vi "Flow Settings Dialog.vi"(8 "error in (no error)":errorcluster, 11 "Flow Module Config In":T1={"GUID"="", "Drop Coords"={"Horizontal"=0, "Vertical"=0}, "Process Name"="", "Settings"={"Cycle Period"=500.0, "Bronkhorst M13"={"VISA resource name"="", "Simulated?"=FALSE}, "Flow Meter Type"="", "Bronkhorst M14"={"VISA resource name"="", "Simulated?"=FALSE}}, "Load Count"=0}) -> (0 "error out":errorcluster, 1 "Cancelled?":bool=TRUE, 2 "UI Refresh Needed?":bool, 3 "Flow Module Config Out":T1={"GUID"="", "Drop Coords"={"Horizontal"=0, "Vertical"=0}, "Process Name"="", "Settings"={"Cycle Period"=500.0, "Bronkhorst M13"={"VISA resource name"="", "Simulated?"=FALSE}, "Flow Meter Type"="", "Bronkhorst M14"={"VISA resource name"="", "Simulated?"=FALSE}}, "Load Count"=0})   [LabVIEW 2018, in "Flow Module.lvlib"]
doc: "Dialog for selecting user specified settings."
uses:
  Flow Module.lvlib
  Feed Module/Controls/Flow Module Settings Cluster.ctl
  Mettler Toledo/Controls/Settings Cluster.ctl
  Feed Module/Controls/Flow Module Config Cluster.ctl
  <vilib>/Utility/miscctls.llb/LVPoint32TypeDef.ctl
  <vilib>/Utility/xml.llb/Write to XML File(string).vi
  Settings/Settings.lvlib
  Bronkhorst M13 Flow Meter/Bronkhorst M13 Flow Meter.lvlib
  Bronkhorst M14 Flow Meter/Bronkhorst M14 Flow Meter.lvlib
  Mettler Toledo/Mettler Toledo.lvlib
panel:
  in  "Module Name":string
  in  "Flow Meter Configuration":T3={"Cycle Period"=500.0, "Bronkhorst M13"={"VISA resource name"="", "Simulated?"=FALSE}, "Flow Meter Type"="Default", "Bronkhorst M14"={"VISA resource name"="", "Simulated?"=FALSE}}
  in  "Cancel Button":bool
  in  "OK Button":bool
  # "Non visible portion of dialog (needed for connector pane)."
  # "Flow Meter Settings"
  # "Flow Meter Settings"
  # "Flow Meter Settings"
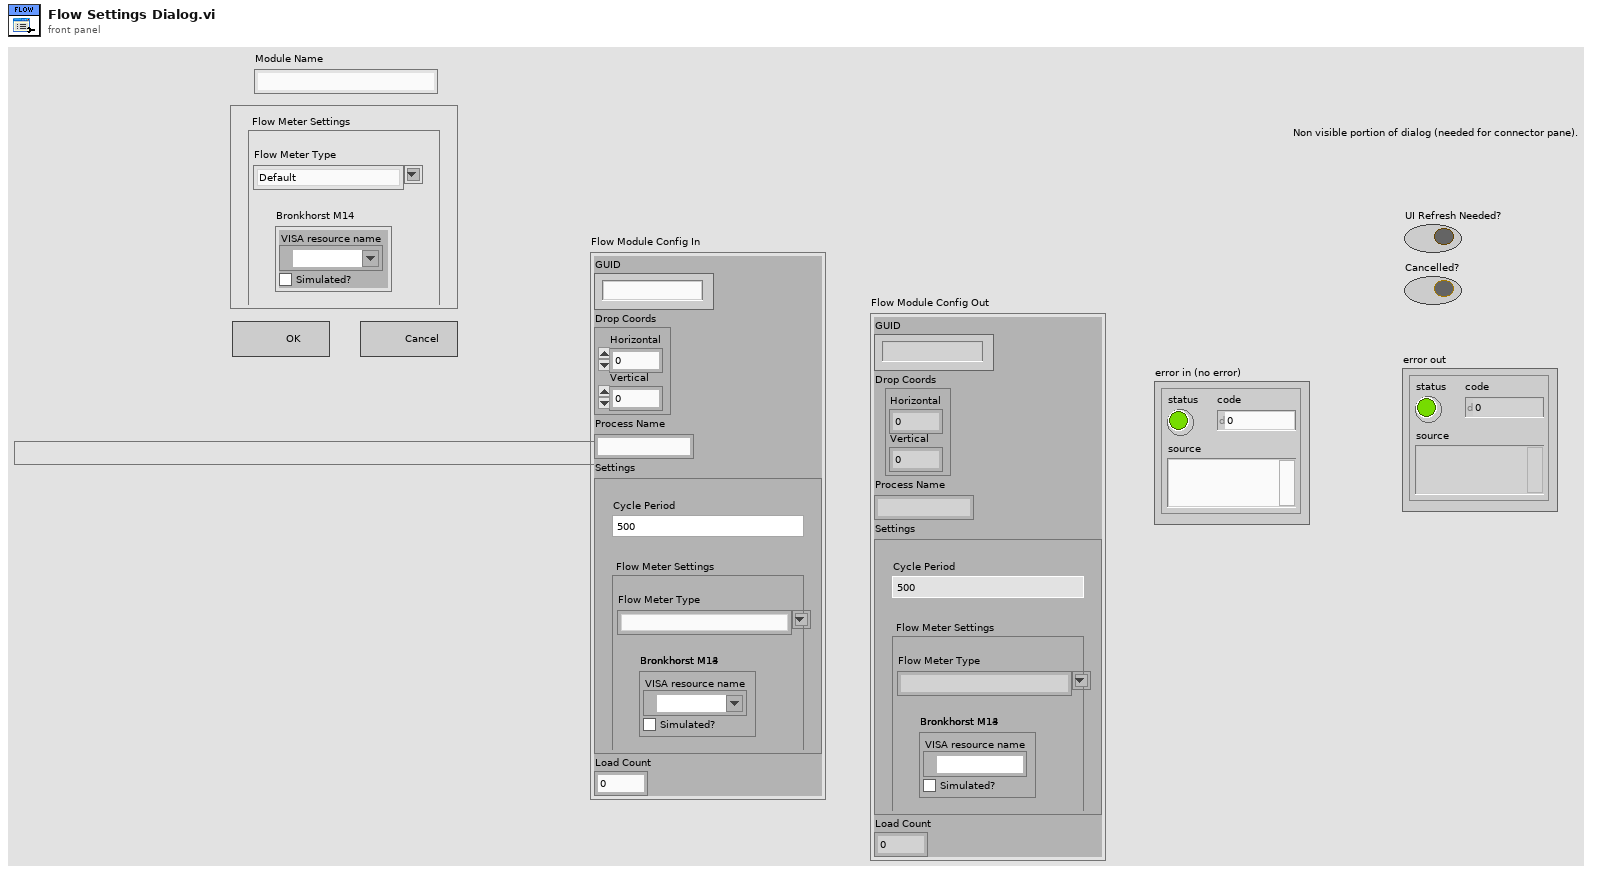
[diagram p1: front panel]
types:
  T1 = typedef "Flow Module.lvlib/Flow Module Config Cluster.ctl" = cluster{"GUID":string, "Drop Coords":T2, "Process Name":string, "Settings":T3, "Load Count":i32}
  T2 = typedef "LVPoint32TypeDef.ctl" = cluster{"Horizontal":i32, "Vertical":i32}
  T3 = typedef "Flow Module.lvlib/Flow Module Settings Cluster.ctl" = cluster{"Cycle Period":dbl, "Bronkhorst M13":T4, "Flow Meter Type":string, "Bronkhorst M14":T4}
  T4 = typedef "Mettler Toledo.lvlib/Settings Cluster.ctl" = cluster{"VISA resource name":refnum<visa-resource-name>, "Simulated?":bool}
  T5 = enum8{"Enabled", "Disabled", "Disabled and Grayed Out"}
  T6 = typedef "Bronkhorst M13 Flow Meter.lvlib/Settings Cluster.ctl" = cluster{"VISA resource name":refnum<visa-resource-name>, "Simulated?":bool}
  T7 = typedef "Bronkhorst M14 Flow Meter.lvlib/Settings Cluster.ctl" = cluster{"VISA resource name":refnum<visa-resource-name>, "Simulated?":bool}
  T8 = cluster{"Cycle Period":dbl, "Bronkhorst M13":T4, "Flow Meter Type":string, "Bronkhorst M14":T4}
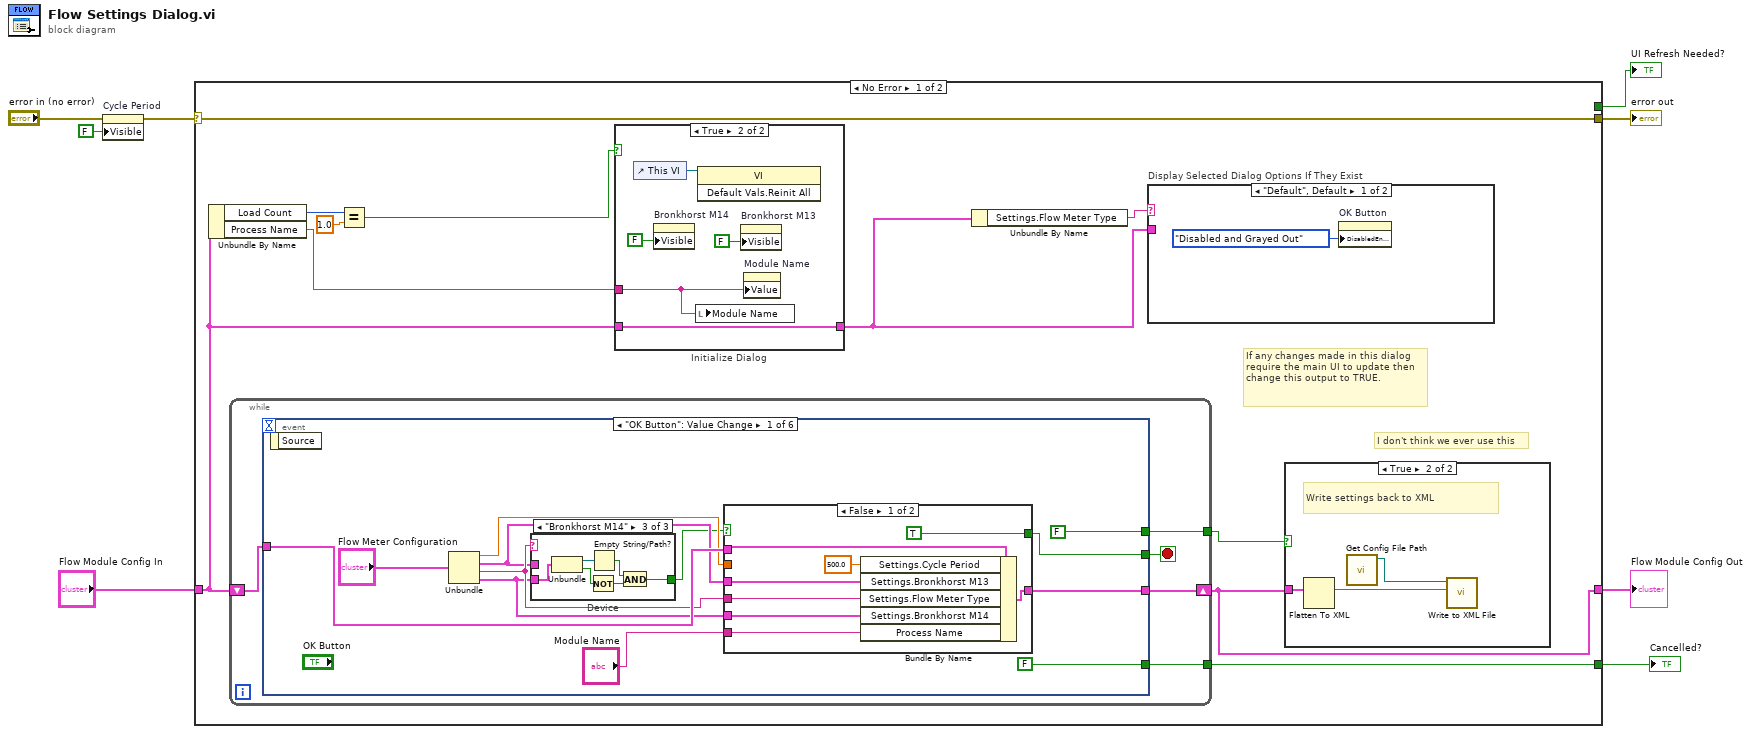
[diagram p0: block diagram]
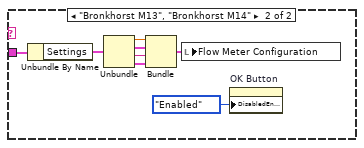
[diagram p2: hidden frame]
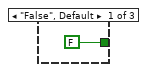
[diagram p4: hidden frame]
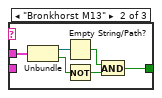
[diagram p5: hidden frame]
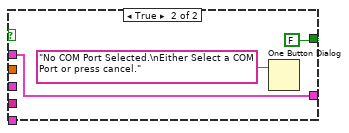
[diagram p6: hidden frame]
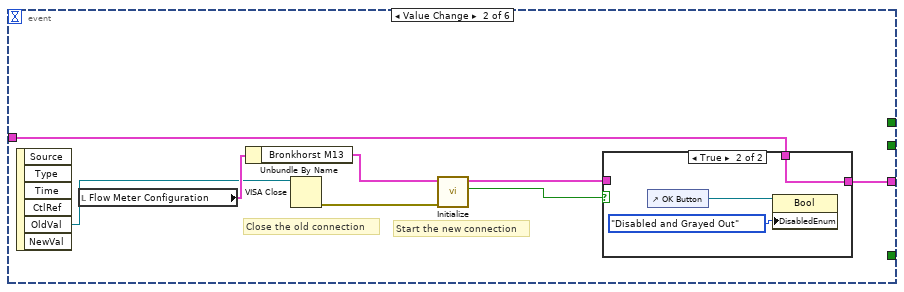
[diagram p7: hidden frame]
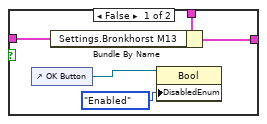
[diagram p8: hidden frame]
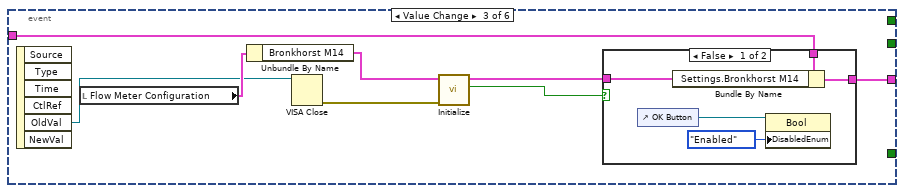
[diagram p9: hidden frame]
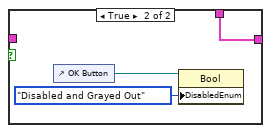
[diagram p10: hidden frame]
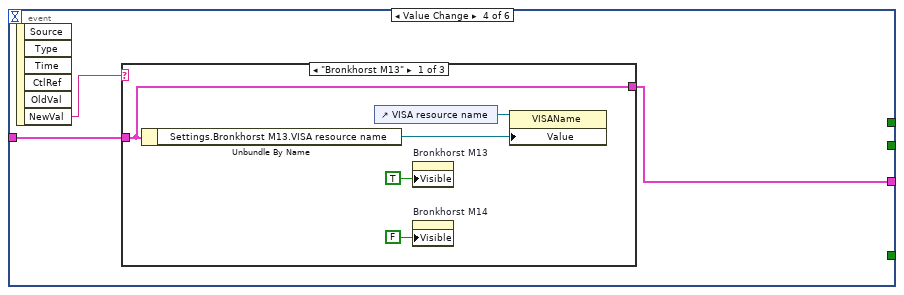
[diagram p11: hidden frame]
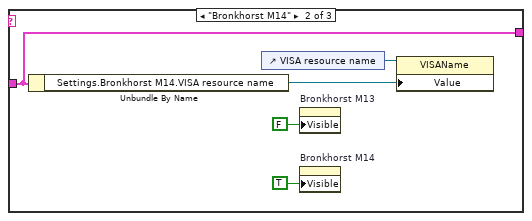
[diagram p12: hidden frame]
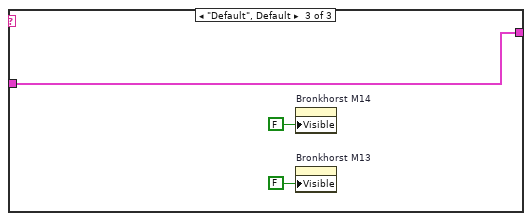
[diagram p13: hidden frame]
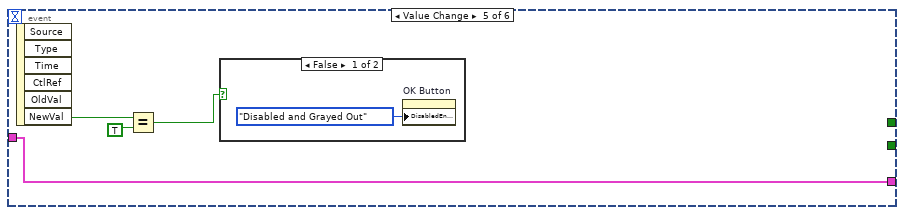
[diagram p14: hidden frame]
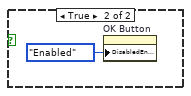
[diagram p15: hidden frame]
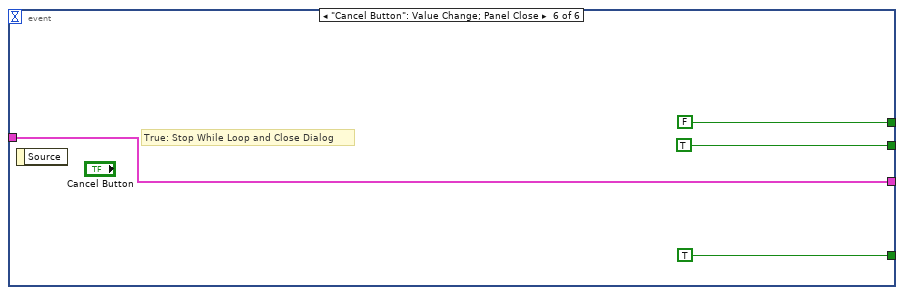
[diagram p16: hidden frame]
diagram:
  n1 = property on="Cycle Period" class="DigNum (strict)"(error in="error in (no error)", "Visible"=FALSE) -> (error out=w1:errorcluster)  [unwired: 1 in, 1 out]
  n2 = case shown="No Error" w1 {
    selector: w1 -> [w20 w140]
    tunnel: [w20 w140] -> w8
    tunnel: "Flow Module Config In" -> [w10 w139]
    tunnel: [w18 w139] -> w4
    tunnel: [FALSE ("UI Refresh Needed?") _] -> w7
    tunnel: [w14 TRUE ("UI Refresh Needed?")] -> w6
    frame No Error {
      # "I don't think we ever use this"
      # "If any changes made in this dialog require the main UI to update then change this output to TRUE."
      n3 = Unbundle By Name(w10) -> ("Load Count"=w17:i32, "Process Name"=w9:string)
      n4 = while {
        tunnel: [w40] -> w15
        tunnel: [w37] -> w14
        shift-right: [w39] -> w18
        shift-left: w10 -> [w36]
        stop <- w38 stop-if-true
        n5 = event shown="[0] \"OK Button\": Value Change" {
          selector: _ -> [_ _ _ _ _ _]
          dyn-events: _ -> [_ _ _ _ _ _]
          timeout: _ -> [_ _ _ _ _ _]
          tunnel: [w50 w82 w98 w110 w128 w134] -> w39
          tunnel: w36 -> [w49 w83 w99 w109 w128 w134]
          tunnel: [FALSE ("UI Refresh Needed?") _ _ _ _ FALSE ("UI Refresh Needed?")] -> w40
          tunnel: [w51 _ _ _ _ TRUE] -> w38
          tunnel: [FALSE ("UI Refresh Needed?") _ _ _ _ TRUE ("UI Refresh Needed?")] -> w37
          event "OK Button": Value Change {
            n6 = event-data() -> ()  [unwired: 1 in, 1 out]
            n7 = Unbundle("Flow Meter Configuration") -> ("Cycle Period"=w47:dbl, "Bronkhorst M13"=w44:T4, "Flow Meter Type"=w45:string, "Bronkhorst M14"=w42:T4)
            n8 = case "Device" shown="\"Bronkhorst M14\"" w45 {
              tunnel: w44 -> [_ w59 _]
              tunnel: [FALSE w54 w61] -> w43
              tunnel: w42 -> [_ _ w60]
              frame "False", Default {
              }
              frame "Bronkhorst M13" {
                n9 = Unbundle(w59) -> ("VISA resource name"=w58:refnum<visa-resource-name>, "Simulated?"=w57:bool)
                n10 = Empty String/Path?(string/path=w58) -> (empty?=w55:bool)
                n11 = Not(x=w57) -> (.not. x?=w56:bool)
                n12 = And(x=w55, y=w56) -> (x .and. y?=w54:bool)
              }
              frame "Bronkhorst M14" {
                n13 = Unbundle(w60) -> ("VISA resource name"=w65:refnum<visa-resource-name>, "Simulated?"=w64:bool)
                n14 = Not(x=w64) -> (.not. x?=w63:bool)
                n15 = Empty String/Path?(string/path=w65) -> (empty?=w62:bool)
                n16 = And(x=w62, y=w63) -> (x .and. y?=w61:bool)
              }
            }
            n17 = case shown="False" w43 {
              tunnel: [TRUE FALSE] -> w51
              tunnel: [w72 w75] -> w50
              tunnel: w49 -> [w71 w75]
              tunnel: w45 -> [w70 _]
              tunnel: w44 -> [w69 _]
              tunnel: w47 -> [_ _]
              tunnel: w42 -> [w68 _]
              tunnel: "Module Name" -> [w66 _]
              frame False {
                n18 = Bundle By Name(cluster=w71, "Settings.Cycle Period"=500.0, "Settings.Bronkhorst M13"=w69, "Settings.Flow Meter Type"=w70, "Settings.Bronkhorst M14"=w68, "Process Name"=w66) -> (w72:T1)
              }
              frame True {
                n19 = One Button Dialog(message="No COM Port Selected.\nEither Select a COM Port or press cancel.") -> ()  [unwired: 1 in, 1 out]
              }
            }
          }
          event Value Change {
            # "Start the new connection"
            # "Close the old connection"
            n20 = event-data() -> ("OldVal"=w78:refnum<visa-resource-name>)  [unwired: 1 in, 5 out]
            n21 = local read "Flow Meter Configuration"() -> (w84:T3)
            n22 = Unbundle By Name(w84) -> ("Bronkhorst M13"=w81:T4)
            n23 = VISA Close(VISA resource name=w78) -> (error out=w79:errorcluster)  [unwired: 1 in]
            n24 = call "Initialize.vi"("error in (no error)"=w79, "Bronkhorst Settings in"=w81) -> ("No Meter Connnected"=w77:bool, "Bronkhorst Settings out"=w80:T6)  [unwired: 7 in, 1 out]
            n25 = case shown="True" w77 {
              tunnel: w83 -> [w89 w92]
              tunnel: [w88 w92] -> w82
              tunnel: w80 -> [w87 _]
              frame False {
                n26 = control-ref of="OK Button"() -> (w85:refnum<vi>)
                n27 = Bundle By Name(cluster=w89, "Settings.Bronkhorst M13"=w87) -> (w88:T1)
                n28 = property class="Bool"(reference=w85, "DisabledEnum"=T5."Enabled" ("Disabled")) -> ()  [unwired: 1 in, 2 out]
              }
              frame True {
                n29 = control-ref of="OK Button"() -> (w90:refnum<vi>)
                n30 = property class="Bool"(reference=w90, "DisabledEnum"=T5."Disabled and Grayed Out" ("Disabled")) -> ()  [unwired: 1 in, 2 out]
              }
            }
          }
          event Value Change {
            n31 = event-data() -> ("OldVal"=w94:refnum<visa-resource-name>)  [unwired: 1 in, 5 out]
            n32 = local read "Flow Meter Configuration"() -> (w100:T3)
            n33 = Unbundle By Name(w100) -> ("Bronkhorst M14"=w97:T4)
            n34 = VISA Close(VISA resource name=w94) -> (error out=w95:errorcluster)  [unwired: 1 in]
            n35 = call "Initialize.vi"("error in (no error)"=w95, "Bronkhorst Settings in"=w97) -> ("No Meter Connected"=w93:bool, "Bronkhorst Settings out"=w96:T7)  [unwired: 7 in, 1 out]
            n36 = case shown="False" w93 {
              tunnel: w99 -> [w105 w108]
              tunnel: [w104 w108] -> w98
              tunnel: w96 -> [w103 _]
              frame False {
                n37 = control-ref of="OK Button"() -> (w102:refnum<vi>)
                n38 = Bundle By Name(cluster=w105, "Settings.Bronkhorst M14"=w103) -> (w104:T1)
                n39 = property class="Bool"(reference=w102, "DisabledEnum"=T5."Enabled" ("Disabled")) -> ()  [unwired: 1 in, 2 out]
              }
              frame True {
                n40 = control-ref of="OK Button"() -> (w107:refnum<vi>)
                n41 = property class="Bool"(reference=w107, "DisabledEnum"=T5."Disabled and Grayed Out" ("Disabled")) -> ()  [unwired: 1 in, 2 out]
              }
            }
          }
          event Value Change {
            n42 = event-data() -> ("NewVal"=w111:string)  [unwired: 1 in, 5 out]
            n43 = case shown="\"Bronkhorst M13\"" w111 {
              tunnel: [w113 w118 w124] -> w110
              tunnel: w109 -> [w113 w118 w124]
              frame "Bronkhorst M13" {
                n44 = Unbundle By Name(w113) -> ("Settings.Bronkhorst M13.VISA resource name"=w116:refnum<visa-resource-name>)
                n45 = control-ref of="VISA resource name"() -> (w114:refnum<vi>)
                n46 = property on="Bronkhorst M13" class="Clust (strict)"("Visible"=TRUE) -> ()  [unwired: 2 in, 2 out]
                n47 = property on="Bronkhorst M14" class="Clust (strict)"("Visible"=FALSE) -> ()  [unwired: 2 in, 2 out]
                n48 = property on="Property Node" class="VISAName"(reference=w114, "Value"=w116) -> ()  [unwired: 1 in, 2 out]
              }
              frame "Bronkhorst M14" {
                n49 = Unbundle By Name(w118) -> ("Settings.Bronkhorst M14.VISA resource name"=w121:refnum<visa-resource-name>)
                n50 = control-ref of="VISA resource name"() -> (w119:refnum<vi>)
                n51 = property on="Bronkhorst M13" class="Clust (strict)"("Visible"=FALSE) -> ()  [unwired: 2 in, 2 out]
                n52 = property on="Bronkhorst M14" class="Clust (strict)"("Visible"=TRUE) -> ()  [unwired: 2 in, 2 out]
                n53 = property on="Property Node" class="VISAName"(reference=w119, "Value"=w121) -> ()  [unwired: 1 in, 2 out]
              }
              frame "Default", Default {
                n54 = property on="Bronkhorst M14" class="Clust (strict)"("Visible"=FALSE) -> ()  [unwired: 2 in, 2 out]
                n55 = property on="Bronkhorst M13" class="Clust (strict)"("Visible"=FALSE) -> ()  [unwired: 2 in, 2 out]
              }
            }
          }
          event Value Change {
            n56 = event-data() -> ("NewVal"=w126:bool)  [unwired: 1 in, 5 out]
            n57 = Equal?(x=w126, y=TRUE) -> (x = y?=w125:bool)
            n58 = case shown="False" w125 {
              frame False {
                n59 = property on="OK Button" class="Bool"("DisabledEnum"=T5."Disabled and Grayed Out" ("Disabled")) -> ()  [unwired: 2 in, 2 out]
              }
              frame True {
                n60 = property on="OK Button" class="Bool"("DisabledEnum"=T5."Enabled" ("Disabled")) -> ()  [unwired: 2 in, 2 out]
              }
            }
          }
          event "Cancel Button": Value Change; Panel Close {
            # "True: Stop While Loop and Close Dialog"
            n61 = event-data() -> ()  [unwired: 1 in, 1 out]
          }
        }
      }
      n62 = Equal?(x=w17, y=1.0) -> (x = y?=w13:bool)
      n63 = case "Initialize Dialog" shown="True" w13 {
        tunnel: w10 -> [w30 w34]
        tunnel: [w30 w34] -> w11
        tunnel: w9 -> [_ w31]
        frame False {
        }
        frame True {
          n64 = control-ref of="This VI"() -> (w35:refnum<vi>)
          n65 = property on="Bronkhorst M14" class="Clust (strict)"("Visible"=FALSE) -> ()  [unwired: 2 in, 2 out]
          n66 = local write "Module Name"(w31) -> ()
          n67 = invoke class="VI" method="Default Vals.Reinit All"(reference=w35) -> ()  [unwired: 2 in, 3 out]
          n68 = property on="Bronkhorst M13" class="Clust (strict)"("Visible"=FALSE) -> ()  [unwired: 2 in, 2 out]
          n69 = property on="Module Name" class="Str"("Value"=w31) -> ()  [unwired: 2 in, 2 out]
        }
      }
      n70 = Unbundle By Name(w11) -> ("Settings.Flow Meter Type"=w12:string)
      n71 = case "Display Selected Dialog Options If They Exist" shown="\"Default\", Default" w12 {
        tunnel: w11 -> [_ w24]
        frame "Default", Default {
          n72 = property on="OK Button" class="Bool"("DisabledEnum"=T5."Disabled and Grayed Out" ("Disabled")) -> ()  [unwired: 2 in, 2 out]
        }
        frame "Bronkhorst M13", "Bronkhorst M14" {
          n73 = Unbundle By Name(w24) -> ("Settings"=w26:T3)
          n74 = Unbundle(w26) -> ("Cycle Period"=w28:dbl, "Bronkhorst M13"=w29:T4, "Flow Meter Type"=w25:string, "Bronkhorst M14"=w23:T4)
          n75 = Bundle("Cycle Period"=w28, "Bronkhorst M13"=w29, "Flow Meter Type"=w25, "Bronkhorst M14"=w23) -> (w27:T8)  [unwired: 1 in]
          n76 = local write "Flow Meter Configuration"(w27) -> ()
          n77 = property on="OK Button" class="Bool"("DisabledEnum"=T5."Enabled" ("Disabled")) -> ()  [unwired: 2 in, 2 out]
        }
      }
      n78 = case shown="True" w15 {
        tunnel: w18 -> [_ w136]
        frame False {
        }
        frame True {
          # "Write settings back to XML"
          n79 = Flatten To XML(anything=w136) -> (xml string=w135:string)
          n80 = call "Get Config File Path.vi"() -> ("XML File Path"=w137:path)  [unwired: 10 in, 1 out]
          n81 = call-poly <vilib>:"Write to XML File.vi"("XML Input"=w135, "XML File Path"=w137) -> ()  [unwired: 7 in, 3 out]
        }
      }
    }
    frame Error {
    }
  }
  "UI Refresh Needed?" <- w7
  "error out" <- w8
  "Cancelled?" <- w6
  "Flow Module Config Out" <- w4
